vi "Motor Loop (Mixed Mode).vi"   [LabVIEW 2009]
uses:
  TypeDefs/Queue TypeDefs/Motor Instruction.ctl
  TypeDefs/Queue TypeDefs/Motor State.ctl
  Remote Control/Motor Command.ctl
  <vilib>/Platform/TimedLoop/XDataNode/XDataNode.xnode
  <vilib>/Platform/TimedLoop/XDataNode/loadlvalarms.vi
  <vilib>/Platform/TimedLoop/XDataNode/timing_clust.ctl
  <vilib>/Platform/TimedLoop/XDataNode/nitl_modes.ctl
  <vilib>/Platform/TimedLoop/XDataNode/wakeup.ctl
  UI Comm/Watchdog Dish Labels.ctl
  Functional Global Variables/Actions for FG's.ctl
  <vilib>/Platform/TimedLoop/XDataNode/XDNodeRunTimeDep.lvlib
types:
  T1 = typedef "Motor Instruction.ctl" = cluster{"Motor State":T2, "Motor Command":T3}
  T2 = typedef "Motor State.ctl" = enum16{"Wait", "Initialize", "Check FET", "Run", "Stop"}
  T3 = typedef "Motor Command.ctl" = cluster{"Speed":i16, "Turn":i16}
  T4 = typedef "XDNodeRunTimeDep.lvlib/timing_clust.ctl" = cluster{"Expected End [f-1]":u64, "Actual End [f-1]":u64, "Finished Late? [f-1]":bool, "Expected End [i-1]":u64, "Actual End [i-1]":u64, "Finished Late? [i-1]":bool, "Expected Start [i]":u64, "Actual Start [i]":u64, "Expected Start [f]":u64, "Actual Start [f]":u64, "Source Name":string, "Structure Name":string, "Period":i64, "Deadline":i64, "Offset":i64, "Start":i64, "Priority":i32, "Timeout":i32, "Mode":T5, "Wakeup Reason":T6, "Error":errorcluster, "Source Type":string, "Secondary Source Type":string, "Global End Time":u64, "Global Start Time":u64, "Frame Duration":u64, "Iteration Duration":u64, "Assigned CPU":i32, "I/O Scan Engine Mode":u32}
  T5 = typedef "XDNodeRunTimeDep.lvlib/nitl_modes.ctl" = enum32{"No Change", "Process missed periods, maintain original phase", "Discard missed periods, maintain original phase", "Process missed periods, ignore original phase", "Discard missed periods, ignore original phase"}
  T6 = typedef "XDNodeRunTimeDep.lvlib/wakeup.ctl" = enum32{"Normal", "Aborted", "Asynchronous wakeup", "Timing source error", "Timed loop error", "Timeout"}
  T7 = typedef "Watchdog Dish Labels.ctl" = enum16{"GPS", "SICK", "Compass", "Cameras", "Motor Controller", "Debug", "RC Receiver"}
  T8 = typedef "Actions for FG's.ctl" = enum16{"Read", "Write"}
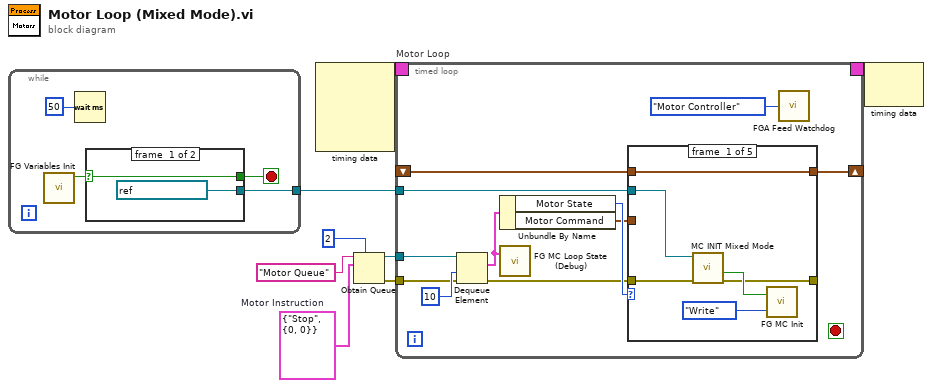
[diagram p0: block diagram]
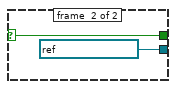
[diagram p2: hidden frame]
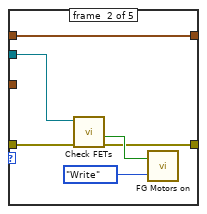
[diagram p3: hidden frame]
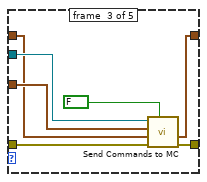
[diagram p4: hidden frame]
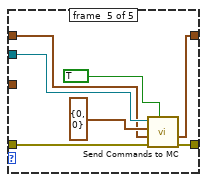
[diagram p6: hidden frame]
diagram:
  w4 = T1 {"Motor State"=enum."Stop", "Motor Command"={"Speed"=0, "Turn"=0}}  # Motor Instruction
  n1 = while {
    tunnel: [w9] -> w6
    stop <- w11 stop-if-true
    n2 = call "FG Variables Init.vi"() -> ("Variables Init out"=w12:bool)  [unwired: 11 in]
    n3 = Wait (ms)(milliseconds to wait=u32 50) -> ()  [unwired: 1 out]
    n4 = case shown="True" w12 {
      selector: w12 -> [w14 w16]
      tunnel: [w14 w16] -> w11
      tunnel: [refnum<visa-resource-name> "RIO0::INSTR" ("MC VISA resource") refnum<visa-resource-name> "ASRL1::INSTR" ("MC VISA resource")] -> w9
      frame #0 {
      }
      frame #1 {
      }
    }
  }
  n5 = node-c288() -> (w8:T4)  [unwired: 4 in]
  n6 = Obtain Queue(max queue size (-1, unlimited)=2, name (unnamed)="Motor Queue", element data type=w4) -> (queue out=w2:refnum<queue>, error out=w1:errorcluster)  [unwired: 2 in, 1 out]
  n7 = timed-loop "Motor Loop" {
    timing: w8 -> [_]
    timing-out: [_] -> w7
    shift-right: [w26] -> _
    shift-left: _ -> [w27]
    tunnel: w6 -> [w25]
    tunnel: w2 -> [w21]
    tunnel: w1 -> [w18]
    stop <- _ stop-if-true
    n8 = Dequeue Element(queue=w21, timeout in ms (-1)=10, error in (no error)=w18) -> (element=w22:T1, error out=w17:errorcluster)  [unwired: 2 out]
    n9 = Unbundle By Name(w22) -> ("Motor State"=w24:T2, "Motor Command"=w23:T3)
    n10 = call "FG MC Loop State (Debug).vi"("Motor Instruction in"=w22) -> ()  [unwired: 1 in, 1 out]
    n11 = case shown="\"Initialize\"" w24 {
      tunnel: w25 -> [w33 w39 w46 _ w55]
      tunnel: w23 -> [_ _ w44 _ _]
      tunnel: w27 -> [w32 w38 w43 w48 w51]
      tunnel: [w32 w38 w42 w48 w52] -> w26
      tunnel: w17 -> [w29 w34 w41 w47 w50]
      tunnel: [w28 w35 w40 w47 w49] -> _
      frame #0 {
        n12 = call "MC INIT Mixed Mode.vi"("error in (no error)"=w29, "MC VISA resource in"=w33) -> ("MC error out"=w28:errorcluster, "MC Init Complete"=w31:bool)  [unwired: 7 in, 1 out]
        n13 = call "FG MC Init.vi"("FG Action"=Actions_for_FG's."Write", "MC Init in"=w31) -> ()  [unwired: 1 out]
      }
      frame #1 {
        n14 = call "Check FETs.vi"("error in (no error)"=w34, "MC VISA resource in"=w39) -> ("error out"=w35:errorcluster, "FETs on?"=w37:bool)  [unwired: 5 in, 3 out]
        n15 = call "FG Motors on.vi"("FG Action"=Actions_for_FG's."Write", "Motors on ? in"=w37) -> ()  [unwired: 1 out]
      }
      frame #2 {
        n16 = call "Send Commands to MC.vi"("Pause Motors"=FALSE, "error in"=w41, "Prev MC cmd"=w43, "Motor Command"=w44, "MC refrence in"=w46) -> ("error out"=w40:errorcluster, "New MC cmd"=w42:cluster{"cmd a":i16, "cmd b":i16})  [unwired: 3 in, 2 out]
      }
      frame #3 {
      }
      frame #4 {
        n17 = call "Send Commands to MC.vi"("Pause Motors"=TRUE, "error in"=w50, "Prev MC cmd"=w51, "Motor Command"=T3 {"Speed"=0, "Turn"=0}, "MC refrence in"=w55) -> ("error out"=w49:errorcluster, "New MC cmd"=w52:cluster{"cmd a":i16, "cmd b":i16})  [unwired: 3 in, 2 out]
      }
    }
    n18 = call "FGA Feed Watchdog.vi"("Watchdog Dish"=Watchdog_Dish_Labels."Motor Controller") -> ()  [unwired: 1 out]
  }
  n19 = node-c288(w7) -> ()  [unwired: 1 out]
